vi "Remove Step at Index.vi"(8 "error in (no error)":errorcluster, 10 "Element":i32, 11 "Loop in":refnum<class "Loop.lvclass">) -> (0 "error out":errorcluster, 3 "Loop out":refnum<class "Loop.lvclass">)   [LabVIEW 2024, in "Ramses Sequencer.lvlib" / "Loop.lvclass"]
uses:
  Loop.lvclass
  Loop.lvclass/Loop.ctl
  Sequence/Sequence.lvclass
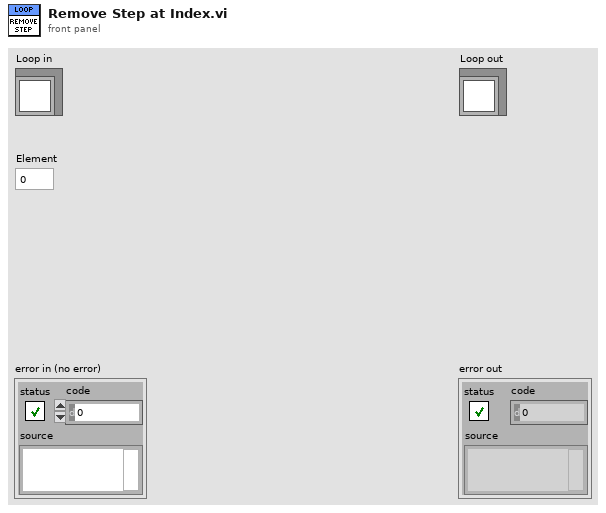
[diagram p1: front panel]
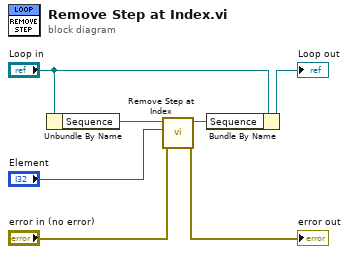
[diagram p0: block diagram]
diagram:
  n1 = Unbundle By Name("Loop in") -> ("Sequence"=w5:refnum<class "Sequence.lvclass">)
  n2 = call "Remove Step at Index.vi"("error in (no error)"="error in (no error)", "Index"="Element", "Sequence in"=w5) -> ("error out"=→"error out":errorcluster, "Sequence out"=w4:refnum<class "Sequence.lvclass">)  [unwired: 7 in]
  n3 = Bundle By Name(cluster="Loop in", "Sequence"=w4) -> (→"Loop out":refnum<class "Loop.lvclass">)
